vi "ep_IIR Cascade Filter.vi"(0 "X":dbl[](array[numeric]), 5 "IIR Filter Cluster":T1 {"Forward Coefficients" format="%.4f"; "Reverse Coefficients" format="%.4f"}, 9 "shift register in":dbl[](array[numeric]), 11 "init/cont (init:F)":bool) -> (4 "Filtered X":dbl[](array[numeric]), 10 "shift register out":dbl[](array[numeric]), 15 "error":i32)   [LabVIEW 2011, in "NI_EP_Power Quality.lvlib"]
uses:
  <vilib>/addons/Electrical Power/PQ/NI_EP_Power Quality.lvlib
  resource/lvanlys.dll
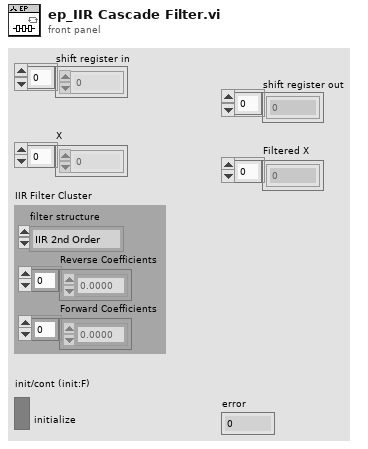
[diagram p1: front panel]
types:
  T1 = cluster{"filter structure":enum32{"IIR 2nd Order", "IIR 4th Order"}, "Reverse Coefficients":dbl[], "Forward Coefficients":dbl[]}
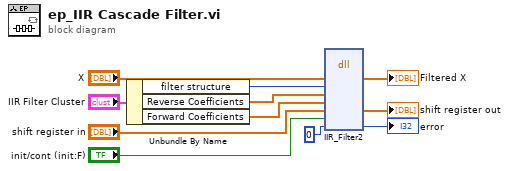
[diagram p0: block diagram]
diagram:
  n1 = Unbundle By Name("IIR Filter Cluster") -> ("filter structure"=w9:enum32{"IIR 2nd Order", "IIR 4th Order"}, "Reverse Coefficients"=w8:dbl[], "Forward Coefficients"=w7:dbl[])
  n2 = dll-call lib="C:/Program Files/National Instruments/LabVIEW 2011/resource/lvanlys.*" fn="IIR_Filter2"("xH"="X", "stage_type"=w9, "aH"=w8, "bH"=w7, "sH"="shift register in", "reset"="init/cont (init:F)", "dsperr"=0) -> ("xH"=→"Filtered X":dbl[], "sH"=→"shift register out":dbl[], "dsperr"=→"error":i32)  [unwired: 8 in, 2 out]
